vi "test_mscu.vi"() -> ()   [LabVIEW 2019, in "MSCU.lvclass"]
uses:
  MSCU.lvclass
panel:
  in  "VISA resource name":refnum<visa-resource-name>
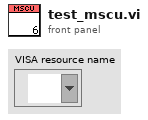
[diagram p1: front panel]
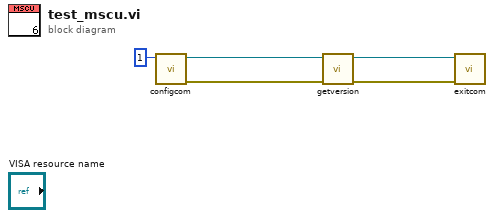
[diagram p0: block diagram]
diagram:
  n1 = call "configcom.vi"("Com port"=1) -> ("error out"=w3:errorcluster, "MSCU"=w4:refnum<class "MSCU.lvclass">)  [unwired: 8 in, 1 out]
  n2 = call "getversion.vi"("error in (no error)"=w3, "MSCU"=w4) -> ("error out"=w2:errorcluster, "MSCU"=w1:refnum<class "MSCU.lvclass">)  [unwired: 6 in, 2 out]
  n3 = call "exitcom.vi"("error in (no error)"=w2, "MSCU"=w1) -> ()  [unwired: 7 in, 3 out]
